vi "Finalize To Settings.vi"(8 "error in (no error)":errorcluster, 11 "UDPlog Thread Configuration in":refnum<class "UDPlog Thread Configuration.lvclass">) -> (0 "error out":errorcluster, 2 "settings":cluster{"key":string, "value":string}[](array[cluster]), 3 "UDPlog Thread Configuration out":refnum<class "UDPlog Thread Configuration.lvclass">)   [LabVIEW 2023, in "UDPlog.lvlib" / "UDPlog Thread Configuration.lvclass"]
uses:
  UDPlog Thread Configuration.lvclass
  UDPlog Thread Configuration.lvclass/UDPlog Thread Configuration.ctl
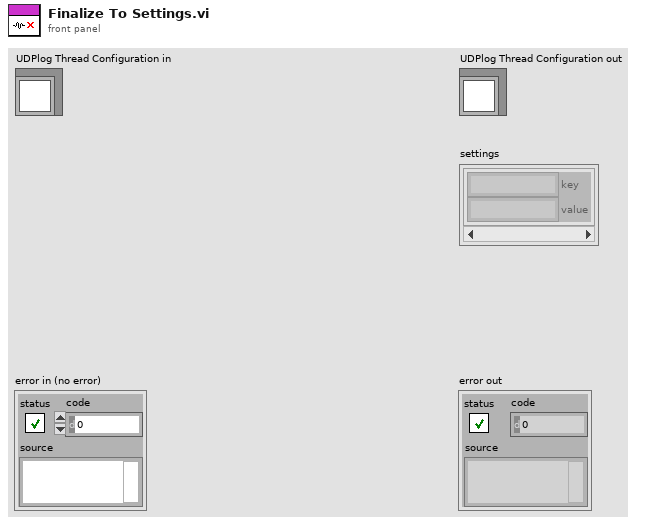
[diagram p1: front panel]
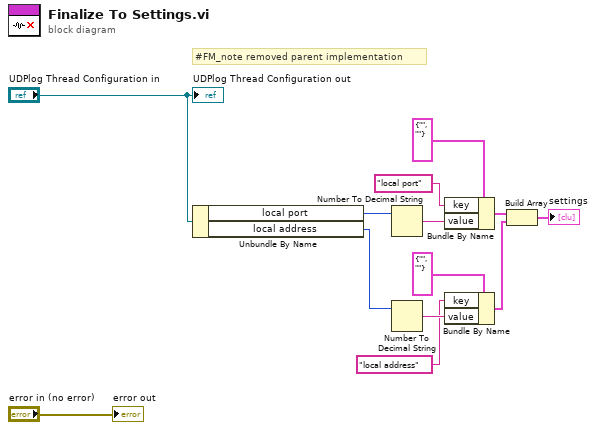
[diagram p0: block diagram]
diagram:
  # "#FM_note removed parent implementation"
  n1 = Unbundle By Name("UDPlog Thread Configuration in") -> ("local port"=w3:u16, "local address"=w2:u32)
  n2 = Number To Decimal String(number=w3) -> (decimal integer string=w5:string)  [unwired: 1 in]
  n3 = Number To Decimal String(number=w2) -> (decimal integer string=w11:string)  [unwired: 1 in]
  n4 = Bundle By Name(cluster=cluster{"key":string, "value":string} {"key"="", "value"=""} ("setting"), "key"="local port", "value"=w5) -> (w10:cluster{"key":string, "value":string})
  n5 = Bundle By Name(cluster=cluster{"key":string, "value":string} {"key"="", "value"=""} ("setting"), "key"="local address", "value"=w11) -> (w9:cluster{"key":string, "value":string})
  n6 = Build Array(w10, w9) -> (→"settings":cluster{"key":string, "value":string}[])
  "error out" <- "error in (no error)"
  "UDPlog Thread Configuration out" <- "UDPlog Thread Configuration in"
